vi "Camera Switcher.vi"(11 "ComboBox in":refnum<vi>) -> ()   [LabVIEW 2018]
uses:
  <vilib>/Rock Robotics/Network Tables/NT Read Boolean.vi
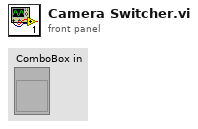
[diagram p1: front panel]
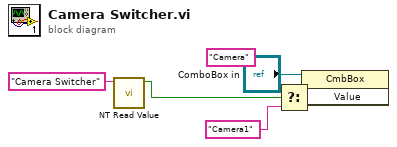
[diagram p0: block diagram]
diagram:
  n1 = call-poly <vilib>:"NT Read Value.vi"("Name"="Camera Switcher") -> ("Boolean"=w5:bool)  [unwired: 9 in, 1 out]
  n2 = Select(t="Camera" ("refnum name"), s=w5, f="Camera1" ("refnum name")) -> (s? t:f=w6:string)
  n3 = property on="Property Node" class="CmbBox"(reference="ComboBox in", "Value"=w6) -> ()  [unwired: 1 in, 2 out]
